vi "np_delay_off (SubVI).vi"(2 "Nose poke in":bool, 3 "npcountin":i16) -> (0 "Nose Poke out":bool, 1 "npcountout":i16)   [LabVIEW 2013]
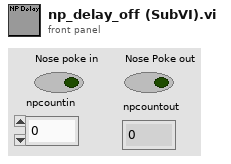
[diagram p1: front panel]
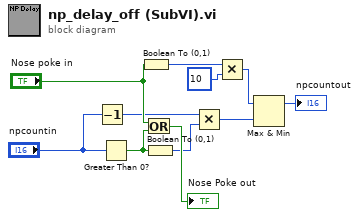
[diagram p0: block diagram]
diagram:
  n1 = Decrement(x="npcountin") -> (x-1=w4:i16)
  n2 = Greater Than 0?(x="npcountin") -> (x > 0?=w1:bool)
  n3 = Boolean To (0,1)(Boolean="Nose poke in") -> (0, 1=w8:i16)
  n4 = Or(x="Nose poke in", y=w1) -> (x .or. y?=→"Nose Poke out":bool)
  n5 = Boolean To (0,1)(Boolean=w1) -> (0, 1=w2:i16)
  n6 = Multiply(x=w4, y=w2) -> (x*y=w3:i16)
  n7 = Multiply(x=w8, y=i16 10) -> (x*y=w6:i16)
  n8 = Max & Min(x=w6, y=w3) -> (max(x,y)=→"npcountout":i16)  [unwired: 1 out]
